vi "AES-KeyExpansion.vi"(8 "error in (no error)":errorcluster, 11 "Key In":u8[](array[numeric]) format="%.0x") -> (0 "error out":errorcluster, 3 "Expanded Key [U8]":u8[](array[numeric]) format="%02x")   [LabVIEW 2012, in "Encryption.lvlib"]
doc: "Expands a Key using AES Key expansion.\n\n(c) Ton Plomp, 2011\nTHIS SOFTWARE IS PROVIDED AS IS, AND ANY WARRANTY IS REJECTED"
uses:
  Encryption.lvlib
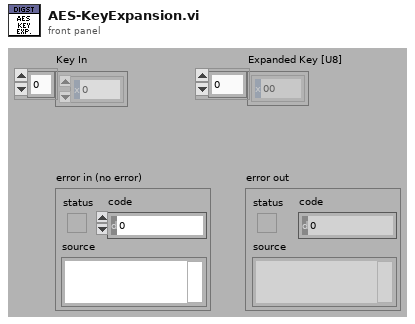
[diagram p1: front panel]
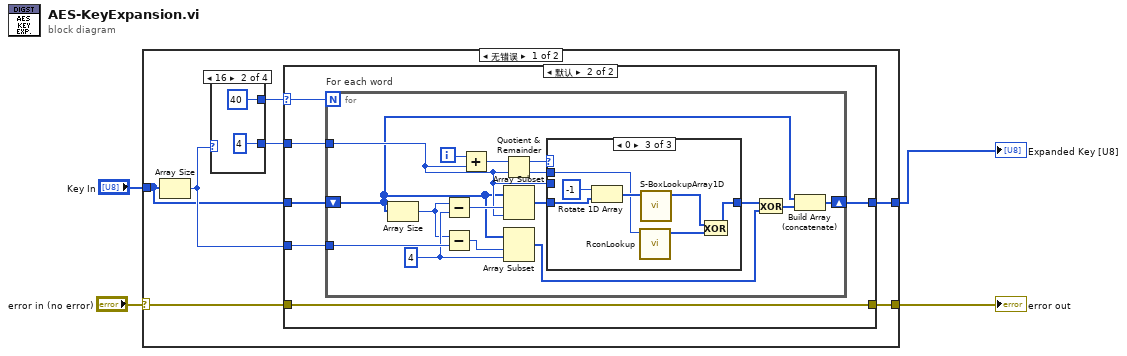
[diagram p0: block diagram]
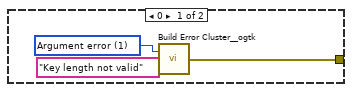
[diagram p2: hidden frame]
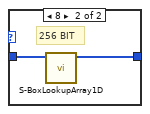
[diagram p5: hidden frame]
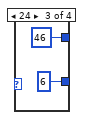
[diagram p7: hidden frame]
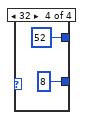
[diagram p8: hidden frame]
diagram:
  n1 = case shown="无错误" "error in (no error)" {
    selector: "error in (no error)" -> [w6 w57]
    tunnel: [w9 _] -> w4
    tunnel: "Key In" -> [w5 _]
    tunnel: [w7 w57] -> w2
    frame No Error {
      n2 = Array Size(array=w5) -> (size(s)=w11:i32)
      n3 = case shown="16" w11 {
        tunnel: [_ 40 46 52] -> w8
        tunnel: [_ 4 6 8] -> w10
        frame 0, Default {
        }
        frame 16 {
        }
        frame 24 {
        }
        frame 32 {
        }
      }
      n4 = case shown="默认" w8 {
        selector: w8 -> [_ w15]
        tunnel: w11 -> [_ w20]
        tunnel: w10 -> [_ w19]
        tunnel: [_ w18] -> w9
        tunnel: w5 -> [_ w17]
        tunnel: w6 -> [_ w16]
        tunnel: [w12 w16] -> w7
        frame 0 {
          w14 = 1 items=["No error", "Argument error", "Memory is full", "Out of zone", "End of file", "File already open", "Generic file I/O error", "File not found", "File permission error", "Disk is full", "Duplicate path", "Too many files open", "System feature not enabled", "Resource file not found", "Cannot add resource", "Resource not found", "Image not found", "Image memory error", "Pen does not exist", "Config type invalid", "Config token not found", "Config parse error", "Config memory error", "Bad external code format", "Bad external code offset", "External code not present", "Null window", "Destroy window error", "Null menu", "Print aborted", "Bad print record", "Print driver error", "Windows error during printing", "Memory error during printing", "Print dialog error", "Generic print error", "Invalid device refnum", "Device not found", "Device parameter error", "Device unit error", "Cannot open device", "Device call aborted", "Generic error", "Cancelled by user", "Object ID too low", "Object ID too high", "Object not in heap", "Unknown heap", "Unknown object (invalid DefProc)", "Unknown object (DefProc not in table)", "Message out of range", "Invalid (null) method", "Unknown message", "Manager call not supported", "Bad address", "Network operation in progress", "Network operation timed out", "Connection is busy", "Network attribute not supported", "Network error", "Address in use", "System out of memory", "Connection aborted", "Connection refused", "Not connected", "Already connected", "Connection closed", "Initialization error (interapplication manager)", "Bad occurrence", "Wait on unbound occurrence handler", "Occurrence queue overflow", "Datalog type conflict", "Unused", "Unrecognized type (interapplication manager)", "Memory corrupt", "Failed to make temporary DLL", "Old CIN version", "Drag socket not found", "Failed to load drop-object", "Failed to register OLE object", "Failed to release OLE object", "Format specifier type mismatch", "Unknown format specifier", "Too few format specifiers", "Too many format specifiers", "Scan failed", "Newer CIN version", "Error converting to variant", "Runtime menu error", "Password tampered", "Variant attribute not found", "Incompatible variant data type", "Event data is not available", "Event Store is not present", "Occurrence is not found", "Event Queue is not created", "Event info is not available", "Refnum passed is NULL", "Error retrieving Class GUID", "Error retrieving CoClass GUID", "Error retrieving TypeLib GUID.", "Bad built application magic bytes.", "Specific driver is different from the specific driver associated with the Logical Name.", "There is no session opened to the class driver.", "Max Error", "MAX - Error with config objects", "MAX - Error loading configuration", "MAX - Group not supported"]
          n5 = call <userlib>:"Build Error Cluster__ogtk.vi"("String to Prepend to source (\"\")"="Key length not valid" ("String to Prepend to source (\"\")"), "code"=w14) -> ("error out"=w12:errorcluster)
        }
        frame Default {
          n6 = for "For each word" {
            N: w15 -> [_]
            shift-right: [w36] -> w18
            shift-left: w17 -> [w23]
            tunnel: w20 -> [w35]
            tunnel: w19 -> [w24]
            i -> [w32]
            w27 = 4 ("y")
            n7 = Array Size(array=w23) -> (size(s)=w21:i32)
            n8 = Subtract(x=w21, y=w27) -> (x-y=w34:i32)
            n9 = Subtract(x=w21, y=w35) -> (x-y=w22:i32)
            n10 = Add(x=w32, y=w24) -> (x+y=w28:i32)
            n11 = Quotient & Remainder(x=w28, y=w24) -> (x-y*floor(x/y)=w33:i32, floor(x/y)=w25:i32)
            n12 = Array Subset(array=w23, index=w34, length=w24) -> (w29:u8[])
            n13 = Array Subset(array=w23, index=w22, length=w27) -> (w31:u8[])
            n14 = case shown="0" w33 {
              tunnel: w29 -> [w37 w38 w49]
              tunnel: [w37 w39 w44] -> w30
              tunnel: w24 -> [_ w40 _]
              tunnel: w25 -> [_ _ w45]
              frame Default {
              }
              frame 4 {
                n15 = case shown="默认" w40 {
                  tunnel: [w41 w42] -> w39
                  tunnel: w38 -> [w41 w43]
                  frame Default {
                  }
                  frame 8 {
                    # "256 BIT"
                    n16 = call "S-BoxLookupArray1D.vi"("In"=w43) -> ("Out"=w42:u8[])  [unwired: 10 in]
                  }
                }
              }
              frame 0 {
                n17 = Rotate 1D Array(1:w49, 2:-1 ("n")) -> (0:w47:u8[])
                n18 = call "RconLookup.vi"("iteration"=w45) -> ("LookUp-Out"=w48:u8[])  [unwired: 10 in]
                n19 = call "S-BoxLookupArray1D.vi"("In"=w47) -> ("Out"=w46:u8[])  [unwired: 10 in]
                n20 = Exclusive Or(1:w48, 2:w46) -> (0:w44:u8[])
              }
            }
            n21 = Exclusive Or(1:w31, 2:w30) -> (0:w26:u8[])
            n22 = Build Array (concatenate)(w23, w26) -> (w36:u8[])
          }
        }
      }
    }
    frame Error {
    }
  }
  "Expanded Key [U8]" <- w4
  "error out" <- w2
